vi "Rename Device.vi"(0 "session in":refnum<k21>, 5 "device":refnum<k21>, 7 "new device name":string, 11 "error in (no error)":errorcluster) -> (4 "session out":refnum<k21>, 15 "error out":errorcluster)   [LabVIEW 2020, in "SLSC.lvlib"]
doc: "Renames the specified <B>device</B> to the <B>new device name</B> on the remote device and in the local configuration file. When renaming a chassis, the hostname of the chassis will be changed on the chassis, but it will not be updated in the local configuration file. After the network is expected to reflect the new hostname, call Add Network Chassis to update the hostname in the local configuration file."
uses:
  <vilib>/SLSC/SLSC.lvlib
  nislsclvapi.dll
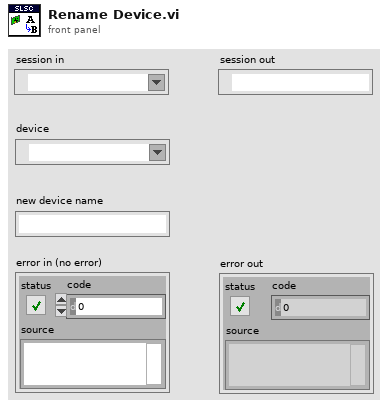
[diagram p1: front panel]
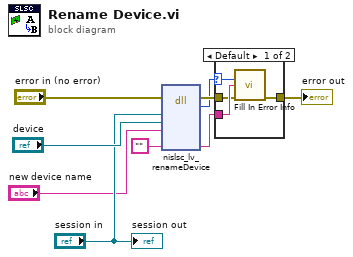
[diagram p0: block diagram]
diagram:
  n1 = dll-call lib="nislsclvapi.*" fn="nislsc_lv_renameDevice"(error in="error in (no error)", "session"="session in", "device"="device", "newDeviceName"="new device name", "extendedErrorInfo"="") -> (error out=w4:errorcluster, "return type"=w3:i32, "extendedErrorInfo"=w5:string)  [unwired: 7 in, 1 out]
  n2 = case shown="Default" w3 {
    selector: w3 -> [w13 _]
    tunnel: w5 -> [w12 _]
    tunnel: w4 -> [w11 w14]
    tunnel: [w10 w14] -> w2
    frame Default {
      n3 = call <vilib>:"Fill In Error Info.vi"("status code"=w13, "extended error info"=w12, "error in"=w11) -> ("error out"=w10:errorcluster)  [unwired: 12 in]
    }
    frame 0 {
    }
  }
  "error out" <- w2
  "session out" <- "session in"
